vi "Loop_SEN.vi"() -> ()   [LabVIEW 2017, in "Dashboard.lvlib"]
uses:
  Dashboard.lvlib
  Shared/TypeDef/Cluster_Encoder_Count.ctl
  Shared/TypeDef/Cluster_Drive_RPM.ctl
  Shared/TypeDef/Cluster_SRX_Amperage.ctl
  Globals/Global_STOP.vi
  Compressor/Globals/GLOBAL_ACT Write_Data_Out.vi
  Globals/Global_CMD_Drive.vi
  WC Drive/Global_ACT Write_Data Out.vi
  Global_SEN Write_Data.vi
  System_Monitoring/Global_SEN Write_Data.vi
  Globals/Global_CMD_Gear.vi
  Compressor/Compressor.lvlib
  WC Drive/WC Drive.lvlib
  System_Monitoring/System_Status.lvlib
panel:
  out "Cycle Time (S)":dbl format="%.3g"
  in  "Target Time(ms)":u32=50
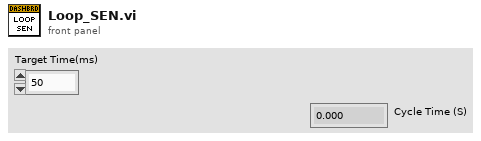
[diagram p1: front panel]
types:
  T1 = cluster{"Target Time(ms)":u32, "Current Time":timestamp, "Previous Time":timestamp, "Cycle Time (S)":dbl, "Num NET Vars":i32}
  T2 = typedef "Cluster_Encoder_Count.ctl" = cluster{"Left Side Encoder":dbl, "Right Side Encoder":dbl}
  T3 = typedef "Cluster_Drive_RPM.ctl" = cluster{"Left Side":dbl, "Right Side":dbl}
  T4 = typedef "Cluster_SRX_Amperage.ctl" = cluster{"Left Back":dbl, "Right Front":dbl, "Right Back":dbl, "Left Front":dbl}
  T5 = typedef "Cluster_Compressor.ctl" = cluster{"Compressor Running":bool, "Compressor Enabled":bool}
  T6 = typedef "CLUSTER_CMD_WC_Drive.ctl" = cluster{"Drive_Mode":T7, "VBus":T8, "Profile":T10}
  T7 = typedef "ENUM_WC_Drive_DriveMode.ctl" = enum16{"Motion Profile", "VBus", "Stop"}
  T8 = typedef "CLUSTER_Drive_ACT Loop_VBus Data.ctl" = cluster{"Drive":T9, "Turbo":bool}
  T9 = typedef "CLUSTER_X and Y.ctl" = cluster{"Steer":dbl, "Throtle":dbl}
  T10 = typedef "CLUSTER_Drive_ACT Loop_Profile Data.ctl" = cluster{"Start":bool}
  T11 = typedef "CLUSTER_Drive_HW_SRX_Status.ctl" = cluster{"Rear Left":T12, "Rear Right":T12, "Front Left":T12, "Front Right":T12}
  T12 = typedef "CLUSTER_4296_SRX_Status.ctl" = cluster{"Status":T13, "Encoder":T14, "PWM ":T15, "Analog":T16, "Limit Switches":T17, "Profile":T18}
  T13 = typedef "CLUSTER_SRX_Status Data.ctl" = cluster{"Module Enabled":bool, "Current Profile Slot Select":dbl, "Brake is Enabled":bool, "Applied Throttle":dbl, "Current":dbl, "Battery Voltage":dbl, "Sticky Fault - Under Voltage":bool, "Temperature (C)":dbl, "Sticky Fault - Over Temp":bool, "CAN Error":errorcluster, "Control 5 Is Supported":bool}
  T14 = typedef "CLUSTER_SRX_Encoder Data.ctl" = cluster{"Closed Loop Error":dbl, "Sensor Position":dbl, "Sensor Velocity":dbl, "Encoder Position":dbl, "Encoder Velocity":dbl, "Encoder Index Count":dbl, "Encoder A Pin State":bool, "Encoder B Pin State":bool, "Encoder Index Pin State":bool, "Pos Div 8":bool, "Vel Div 4":bool}
  T15 = typedef "CLUSTER_SRX_PWM Data.ctl" = cluster{"Closed Loop Error":dbl, "Pulse Width Position":i32, "Pulse Width Velocity":i32, "Pulse Width Rise To Rise (us)":i32, "Pulse Width Rise To Fall (us)":i32}
  T16 = typedef "CLUSTER_SRX_Analog Data.ctl" = cluster{"Closed Loop Error":dbl, "Analog In":dbl, "Analog In Velocity":dbl}
  T17 = typedef "CLUSTER_SRX_Limit Switch Data.ctl" = cluster{"Forward Limit Switch Closed":bool, "Reverse Limit Switch Closed":bool, "Sticky Fault - Forward Limit":bool, "Sticky Fault - Reverse Limit":bool, "Sticky Fault - Forward Soft Limit":bool, "Sticky Fault - Reverse Soft Limit":bool}
  T18 = typedef "CLUSTER_SRX_Profile Data.ctl" = cluster{"Mot Prof Active Is Under Run":bool, "Mot Prof Active Has Under Run":bool, "Mot Prof Active Is Last":bool, "Mot Prof Active Velocity Only":bool, "Mot Prof Active Is Valid":bool, "Mot Prof Buffer Is Full":bool, "Mot Prof Active Profile Slot Select":i32, "Mot Prof NextID":i32, "Mot Prof Count":i32, "Mot Prof Active Velocity":dbl, "Mot Prof Active Position":dbl, "Mot Prof Output Enable":i32}
  T19 = typedef "CLUSTER_Drive_Motion Profile Arrays.ctl" = cluster{"Left":T20[], "Right":T20[]}
  T20 = typedef "CLUSTER_Drive_Point Specification.ctl" = cluster{"Position":dbl, "Velocity":dbl, "headingDeg":dbl, "Duration in ms":i32}
  T21 = typedef "CLUSTER_RoboRio_Status.ctl" = cluster{"RoboRio Faults":T22, "RIO inpt vol (V)":dbl, "RIO inpt cur (A)":dbl, "RoboRio Rails":T23}
  T22 = typedef "CLUSTER_RoboRio_Faults.ctl" = cluster{"Inpt. V. Brn. Out":bool, "3.3V Usr Rail Shrt.":bool, "5 V Usr Rail Shrt.":bool, "6 V Usr. Rail Shrt.":bool, "5V Usr. Rail Brn. Out":bool}
  T23 = typedef "CLUSTER_RoboRio_Rails.ctl" = cluster{"3.3 Volt":T24, "5 Volt":T24, "6 Volt":T24}
  T24 = typedef "CLUSTER_RoboRio_SingleRail.ctl" = cluster{"Vol.  (V)":dbl, "Cur. (A)":dbl}
  T25 = typedef "CLUSTER_PCM_Status.ctl" = cluster{"Current (A)":dbl, "All Solenoid Faults":bool[], "Input Voltage":dbl, "Solenoid Voltage":dbl, "Comp. Fault":bool}
  T26 = typedef "CLUSTER_PDP_Status.ctl" = cluster{"PDP Faults":T27, "All Currents (A)":dbl[], "Energy (J)":dbl, "Power (W)":dbl, "Voltage (V)":dbl}
  T27 = typedef "CLUSTER_PDP_Faults.ctl" = cluster{"Current Faults":bool[], "Batt V Fault":bool, "Temp Fault":bool, "HW Fault":bool}
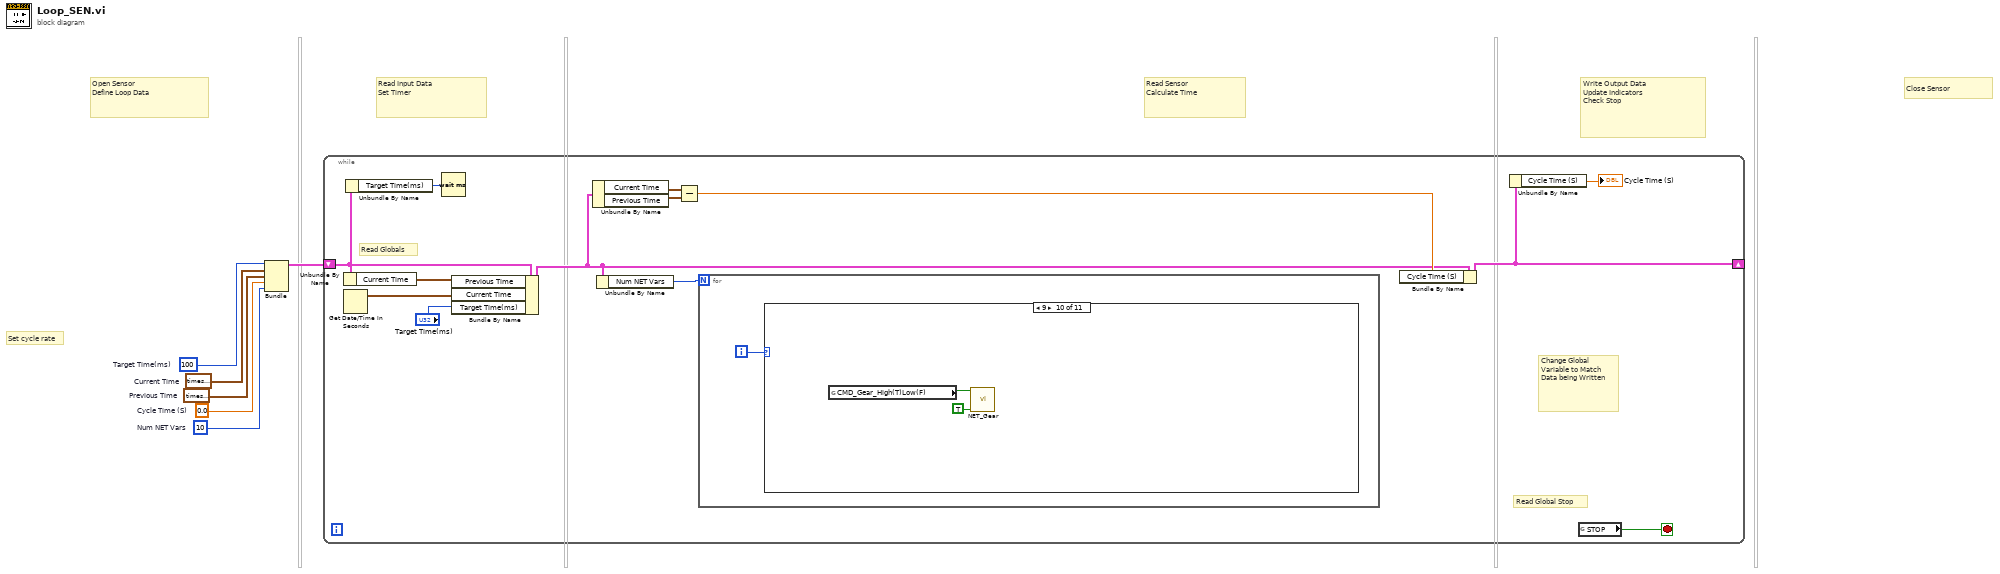
[diagram p0: block diagram]
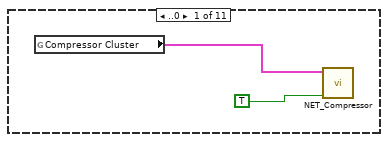
[diagram p2: hidden frame]
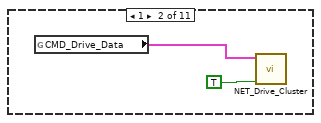
[diagram p3: hidden frame]
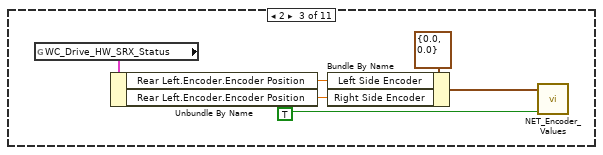
[diagram p4: hidden frame]
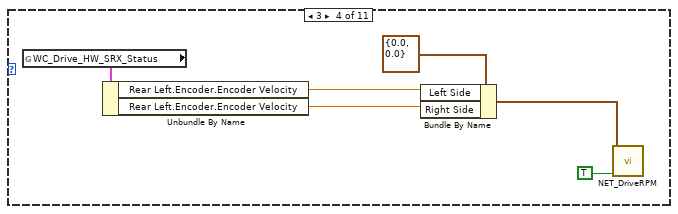
[diagram p5: hidden frame]
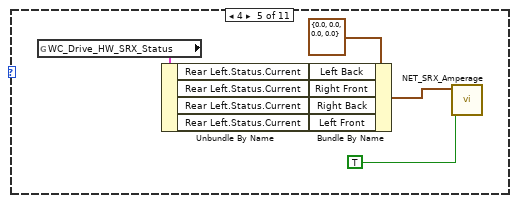
[diagram p6: hidden frame]
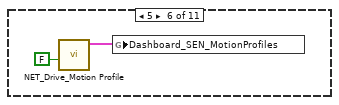
[diagram p7: hidden frame]
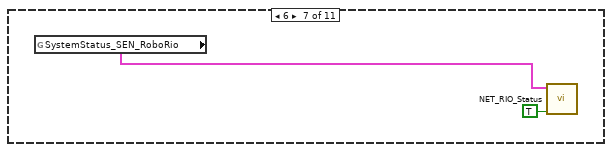
[diagram p8: hidden frame]
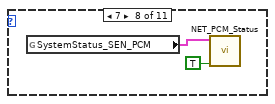
[diagram p9: hidden frame]
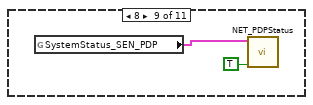
[diagram p10: hidden frame]
diagram:
  w1 = 10  # Num NET Vars
  w2 = 0.0  # Cycle Time (S)
  w6 = timestamp(0 s since 1904-01-01)  # Previous Time
  w5 = timestamp(0 s since 1904-01-01)  # Current Time
  w4 = u32 100  # Target Time(ms)
  # "Close Sensor"
  # "Write Output Data\nUpdate Indicators\nCheck Stop"
  # "Read Sensor\nCalculate Time"
  # "Read Input Data\nSet Timer"
  # "Open Sensor\nDefine Loop Data"
  # "Set cycle rate"
  n1 = Bundle("Target Time(ms)"=w4, "Current Time"=w5, "Previous Time"=w6, "Cycle Time (S)"=w2, "Num NET Vars"=w1) -> (w3:T1)  [unwired: 1 in]
  n2 = while {
    shift-right: [w11] -> _
    shift-left: w3 -> [w13]
    stop <- w19 stop-if-true
    # "Change Global\nVariable to Match\nData being Written"
    # "Read Globals"
    # "Read Global Stop"
    n3 = Unbundle By Name(w13) -> ("Current Time"=w17:timestamp)
    n4 = Get Date/Time In Seconds() -> (seconds since 1Jan1904=w18:timestamp)
    n5 = Unbundle By Name(w13) -> ("Target Time(ms)"=w12:u32)
    n6 = Wait (ms)(milliseconds to wait=w12) -> ()  [unwired: 1 out]
    n7 = Bundle By Name(cluster=w13, "Previous Time"=w17, "Current Time"=w18, "Target Time(ms)"="Target Time(ms)") -> (w8:T1)
    n8 = Unbundle By Name(w8) -> ("Current Time"=w16:timestamp, "Previous Time"=w15:timestamp)
    n9 = Unbundle By Name(w8) -> ("Num NET Vars"=w7:i32)
    n10 = Subtract(x=w16, y=w15) -> (x-y=w9:dbl)
    n11 = for {
      N: w7 -> [_]
      i -> [w20]
      n12 = case shown="9" w20 {
        frame ..0 {
          n13 = global read "GLOBAL_ACT Write_Data_Out.vi" "Compressor Cluster"() -> (w21:T5)
          n14 = call "NET_Compressor.vi"("Read(F) Write(T)"=TRUE, "Compressor  In"=w21) -> ()  [unwired: 9 in, 1 out]
        }
        frame 1 {
          n15 = global read "Global_CMD_Drive.vi" "CMD_Drive_Data"() -> (w23:T6)
          n16 = call "NET_Drive_Cluster.vi"("Read(F) Write(T)"=TRUE, "CMD_DriveCluster"=w23) -> ()  [unwired: 9 in, 1 out]
        }
        frame 2 {
          n17 = global read "Global_ACT Write_Data Out.vi" "WC_Drive_HW_SRX_Status"() -> (w29:T11)
          n18 = Unbundle By Name(w29) -> ("Rear Left.Encoder.Encoder Position"=w28:dbl, "Rear Left.Encoder.Encoder Position"=w27:dbl)
          n19 = Bundle By Name(cluster=T2 {"Left Side Encoder"=0.0, "Right Side Encoder"=0.0} ("Encoder Counts 2"), "Left Side Encoder"=w28, "Right Side Encoder"=w27) -> (w25:T2)
          n20 = call "NET_Encoder_Values.vi"("Read(F) Write(T)"=TRUE, "Encoder Counts"=w25) -> ()  [unwired: 9 in, 1 out]
        }
        frame 3 {
          n21 = global read "Global_ACT Write_Data Out.vi" "WC_Drive_HW_SRX_Status"() -> (w35:T11)
          n22 = Unbundle By Name(w35) -> ("Rear Left.Encoder.Encoder Velocity"=w32:dbl, "Rear Left.Encoder.Encoder Velocity"=w31:dbl)
          n23 = Bundle By Name(cluster=T3 {"Left Side"=0.0, "Right Side"=0.0} ("Drive Encoder Vel"), "Left Side"=w32, "Right Side"=w31) -> (w33:T3)
          n24 = call "NET_DriveRPM.vi"("Read(F) Write(T)"=TRUE, "Drive Encoder Vel"=w33) -> ()  [unwired: 9 in, 1 out]
        }
        frame 4 {
          n25 = global read "Global_ACT Write_Data Out.vi" "WC_Drive_HW_SRX_Status"() -> (w43:T11)
          n26 = Unbundle By Name(w43) -> ("Rear Left.Status.Current"=w42:dbl, "Rear Left.Status.Current"=w41:dbl, "Rear Left.Status.Current"=w40:dbl, "Rear Left.Status.Current"=w39:dbl)
          n27 = Bundle By Name(cluster=T4 {"Left Back"=0.0, "Right Front"=0.0, "Right Back"=0.0, "Left Front"=0.0} ("SRX_Amp_Cluster"), "Left Back"=w42, "Right Front"=w41, "Right Back"=w40, "Left Front"=w39) -> (w38:T4)
          n28 = call "NET_SRX_Amperage.vi"("Read(F) Write(T)"=TRUE, "SRX_Amp_Cluster"=w38) -> ()  [unwired: 9 in, 1 out]
        }
        frame 5 {
          n29 = call "NET_Drive_Motion Profile.vi"("Read(F) Write(T)"=FALSE) -> ("Motion Profile Out"=w46:T19)  [unwired: 9 in, 1 out]
          n30 = global write "Global_SEN Write_Data.vi" "Dashboard_SEN_MotionProfiles"(w46) -> ()
        }
        frame 6 {
          n31 = global read "Global_SEN Write_Data.vi" "SystemStatus_SEN_RoboRio"() -> (w47:T21)
          n32 = call "NET_RIO_Status.vi"("Read(F) Write(T)"=TRUE, "RoboRio Status In"=w47) -> ()  [unwired: 9 in, 1 out]
        }
        frame 7 {
          n33 = global read "Global_SEN Write_Data.vi" "SystemStatus_SEN_PCM"() -> (w50:T25)
          n34 = call "NET_PCM_Status.vi"("Read(F) Write(T)"=TRUE, "PCM_Status_In"=w50) -> ()  [unwired: 9 in, 1 out]
        }
        frame 8 {
          n35 = global read "Global_SEN Write_Data.vi" "SystemStatus_SEN_PDP"() -> (w52:T26)
          n36 = call "NET_PDPStatus.vi"("Read(F) Write(T)"=TRUE, "PDP_Status_In"=w52) -> ()  [unwired: 9 in, 1 out]
        }
        frame 9 {
          n37 = global read "Global_CMD_Gear.vi" "CMD_Gear_High(T)Low(F)"() -> (w53:bool)
          n38 = call "NET_Gear.vi"("Read(F) Write(T)"=TRUE, "High Gear In"=w53) -> ()  [unwired: 9 in, 1 out]
        }
        frame 10.. {
        }
      }
    }
    n39 = Bundle By Name(cluster=w8, "Cycle Time (S)"=w9) -> (w11:T1)
    n40 = Unbundle By Name(w11) -> ("Cycle Time (S)"=→"Cycle Time (S)":dbl)
    n41 = global read "Global_STOP.vi" "STOP"() -> (w19:bool)
  }
